vi "Minimum Jerk Trajectory.vi"(8 "total time":dbl, 9 "total length":dbl, 11 "t (sec)":dbl) -> (1 "In Range?":bool, 3 "ref_x (mm)":dbl)   [LabVIEW 2021]
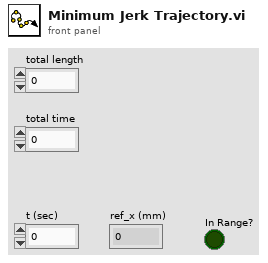
[diagram p1: front panel]
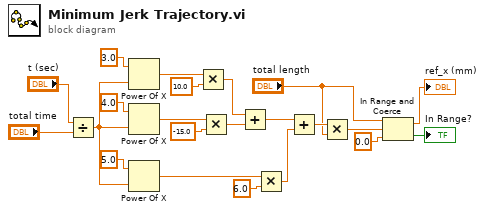
[diagram p0: block diagram]
diagram:
  n1 = Divide(x="t (sec)", y="total time") -> (x/y=w7:dbl)
  n2 = Power Of X(1:w7, 2:3.0 ("y")) -> (0:w11:dbl)
  n3 = Power Of X(1:w7, 2:4.0 ("y")) -> (0:w19:dbl)
  n4 = Power Of X(1:w7, 2:5.0 ("y")) -> (0:w18:dbl)
  n5 = Multiply(x=w11, y=10.0) -> (x*y=w15:dbl)
  n6 = Multiply(x=w19, y=-15.0) -> (x*y=w20:dbl)
  n7 = Add(x=w15, y=w20) -> (x+y=w22:dbl)
  n8 = Multiply(x=w18, y=6.0) -> (x*y=w21:dbl)
  n9 = Add(x=w22, y=w21) -> (x+y=w6:dbl)
  n10 = Multiply(x=w6, y="total length") -> (x*y=w4:dbl)
  n11 = In Range and Coerce(upper limit="total length", x=w4, lower limit=0.0) -> (coerced(x)=→"ref_x (mm)":dbl, In Range?=→"In Range?":bool)
